vi "Multiple Registration - Unregister.vi"() -> ()   [LabVIEW 2011]
panel:
  in  "Unregister 3":bool
  in  "Unregister 1":bool
  out "Iteration Count #3":i32
  out "Iteration Count #2":i32
  out "Iteration Count #1":i32
  in  "Unregister 2":bool
  out "Process 3 Event #":i32
  out "Process 2 Event #":i32
  out "Process 1 Event #":i32
  in  "Generate Event":bool
  out "Time Process 3 was Stopped":timestamp
  out "Process 3":timestamp
  out "Time Process 2 was Stopped":timestamp
  out "Process 2":timestamp
  out "Time Process 1 was Stopped":timestamp
  in  "stop":bool
  out "Process 1":timestamp
  # "Loop\nIteration\nCount"
  # "Event\nNumber"
  # "User Event Data"
  # "Time Process was stopped"
  # "Process 1"
  # "Process 2"
  # "Process 3"
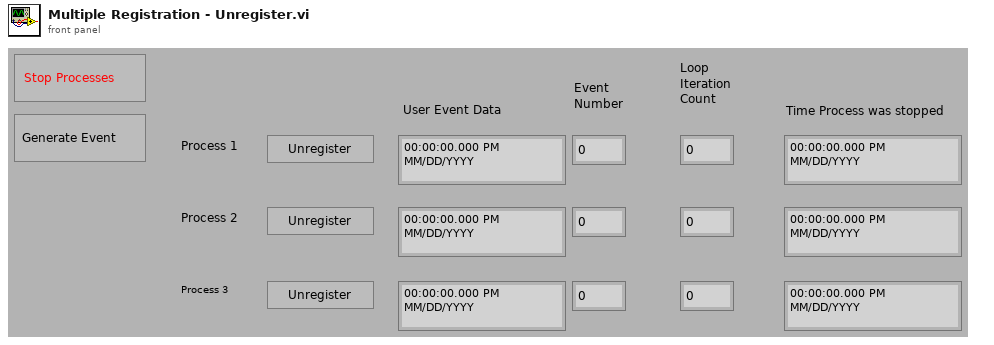
[diagram p1: front panel]
types:
  T1 = cluster{"Event Number":i32, "Event Time":timestamp}
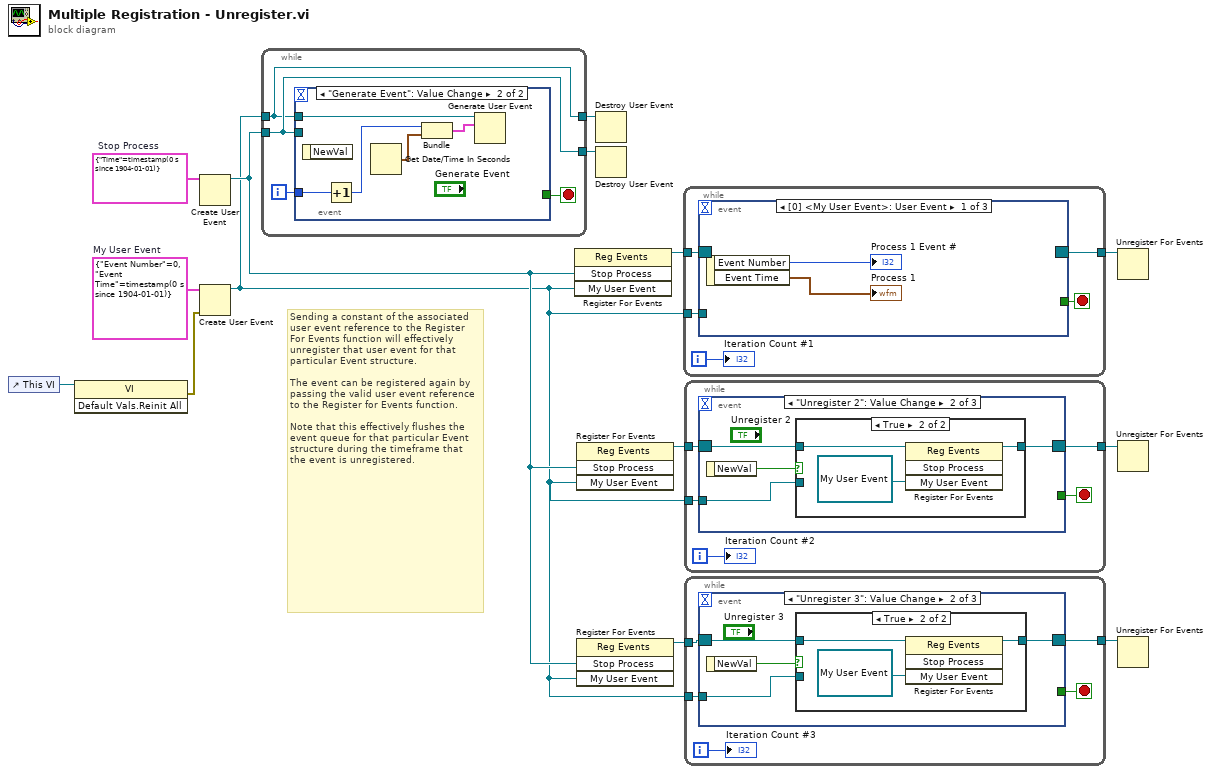
[diagram p0: block diagram]
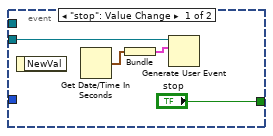
[diagram p2: hidden frame]
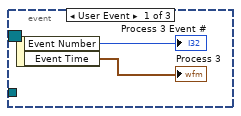
[diagram p3: hidden frame]
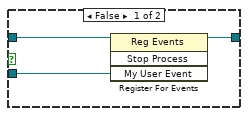
[diagram p4: hidden frame]
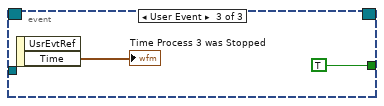
[diagram p5: hidden frame]
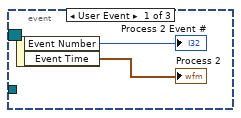
[diagram p6: hidden frame]
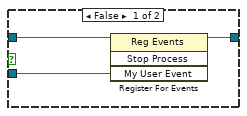
[diagram p7: hidden frame]
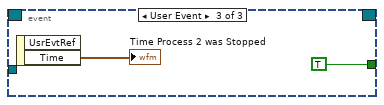
[diagram p8: hidden frame]
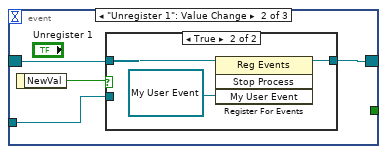
[diagram p9: hidden frame]
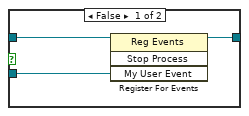
[diagram p10: hidden frame]
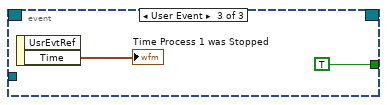
[diagram p11: hidden frame]
diagram:
  w9 = T1 {"Event Number"=0, "Event Time"=timestamp(0 s since 1904-01-01)}  # My User Event
  w14 = cluster{"Time":timestamp} {"Time"=timestamp(0 s since 1904-01-01)}  # Stop Process
  # "Sending a constant of the associated user event reference to the Register For Events function will effectively unregister that user event for that particular Event structure.\n\nThe event can be registered again by passing the valid user event reference to the Register for Events function.\n\nNote that this effectively flushes the event queue for that particular Event structure during the timeframe that the event is unregistered."
  n1 = control-ref of="This VI"() -> (w2:refnum<vi>)
  n2 = invoke class="VI" method="Default Vals.Reinit All"(reference=w2) -> (error out=w1:errorcluster)  [unwired: 2 in, 2 out]
  n3 = Create User Event(user event datatype=w14) -> (user event=w10:refnum<user-event>)  [unwired: 1 in, 1 out]
  n4 = Create User Event(user event datatype=w9, error in=w1) -> (user event=w8:refnum<user-event>)  [unwired: 1 out]
  n5 = while {
    tunnel: w10 -> [w16]
    tunnel: w8 -> [w15]
    tunnel: [w15] -> w7
    tunnel: [w16] -> w6
    i -> [w17]
    stop <- w18 stop-if-true
    n6 = event shown="[1] \"Generate Event\": Value Change" {
      selector: _ -> [_ _]
      dyn-events: _ -> [_ _]
      timeout: _ -> [_ _]
      tunnel: w16 -> [w22 _]
      tunnel: ["stop" _] -> w18
      tunnel: w15 -> [_ w27]
      tunnel: w17 -> [_ w26]
      event "stop": Value Change {
        n7 = event-data() -> ()  [unwired: 1 in, 1 out]
        n8 = Get Date/Time In Seconds() -> (seconds since 1Jan1904=w21:timestamp)
        n9 = Bundle("seconds since 1Jan1904"=w21) -> (w20:cluster{"seconds since 1Jan1904":timestamp})  [unwired: 1 in]
        n10 = Generate User Event(user event=w22, event data cluster=w20) -> ()  [unwired: 1 in, 2 out]
      }
      event "Generate Event": Value Change {
        n11 = event-data() -> ()  [unwired: 1 in, 1 out]
        n12 = Increment(x=w26) -> (x+1=w23:i32)
        n13 = Get Date/Time In Seconds() -> (seconds since 1Jan1904=w25:timestamp)
        n14 = Bundle(w23, "seconds since 1Jan1904"=w25) -> (w24:cluster{i32, "seconds since 1Jan1904":timestamp})  [unwired: 1 in]
        n15 = Generate User Event(user event=w27, event data cluster=w24) -> ()  [unwired: 1 in, 2 out]
      }
    }
  }
  n16 = register-events(w10, w8) -> (reference out=w13:refnum<event-registration>)  [unwired: 2 in, 1 out]
  n17 = register-events(w10, w8) -> (reference out=w12:refnum<event-registration>)  [unwired: 2 in, 1 out]
  n18 = register-events(w10, w8) -> (reference out=w11:refnum<event-registration>)  [unwired: 2 in, 1 out]
  n19 = Destroy User Event(user event=w7) -> ()  [unwired: 1 in, 1 out]
  n20 = Destroy User Event(user event=w6) -> ()  [unwired: 1 in, 1 out]
  n21 = while {
    tunnel: w13 -> [w32]
    tunnel: w8 -> [w29]
    tunnel: [w28] -> w5
    i -> [w30]
    stop <- w31 stop-if-true
    n22 = event shown="[0] <My User Event>: User Event" {
      selector: w32 -> [_ w37 _]
      dyn-events: [_ w36 _] -> w28
      timeout: _ -> [_ _ _]
      tunnel: [_ _ TRUE] -> w31
      tunnel: w29 -> [_ w38 _]
      event User Event {
        n23 = event-data() -> ("Event Number"=→"Process 1 Event #":i32, "Event Time"=→"Process 1":timestamp)  [unwired: 1 in]
      }
      event "Unregister 1": Value Change {
        n24 = event-data() -> ("NewVal"=w35:bool)  [unwired: 1 in]
        n25 = case shown="True" w35 {
          tunnel: w37 -> [w39 w44]
          tunnel: w38 -> [w41 _]
          tunnel: [w40 w43] -> w36
          frame False {
            n26 = register-events(reference=w39, w41) -> (reference out=w40:refnum<event-registration>)  [unwired: 2 in, 1 out]
          }
          frame True {
            n27 = register-events(reference=w44, refnum<user-event> refnum ("event source")) -> (reference out=w43:refnum<event-registration>)  [unwired: 2 in, 1 out]
          }
        }
      }
      event User Event {
        n28 = event-data() -> ("Time"=→"Time Process 1 was Stopped":timestamp)  [unwired: 1 in, 1 out]
      }
    }
    "Iteration Count #1" <- w30
  }
  n29 = while {
    tunnel: w12 -> [w51]
    tunnel: w8 -> [w49]
    tunnel: [w47] -> w4
    i -> [w48]
    stop <- w50 stop-if-true
    n30 = event shown="[1] \"Unregister 2\": Value Change" {
      selector: w51 -> [_ w57 _]
      dyn-events: [_ w54 _] -> w47
      timeout: _ -> [_ _ _]
      tunnel: [_ _ TRUE] -> w50
      tunnel: w49 -> [_ w55 _]
      event User Event {
        n31 = event-data() -> ("Event Number"=→"Process 2 Event #":i32, "Event Time"=→"Process 2":timestamp)  [unwired: 1 in]
      }
      event "Unregister 2": Value Change {
        n32 = event-data() -> ("NewVal"=w56:bool)  [unwired: 1 in]
        n33 = case shown="True" w56 {
          tunnel: w57 -> [w58 w63]
          tunnel: w55 -> [w60 _]
          tunnel: [w59 w62] -> w54
          frame False {
            n34 = register-events(reference=w58, w60) -> (reference out=w59:refnum<event-registration>)  [unwired: 2 in, 1 out]
          }
          frame True {
            n35 = register-events(reference=w63, refnum<user-event> refnum ("event source")) -> (reference out=w62:refnum<event-registration>)  [unwired: 2 in, 1 out]
          }
        }
      }
      event User Event {
        n36 = event-data() -> ("Time"=→"Time Process 2 was Stopped":timestamp)  [unwired: 1 in, 1 out]
      }
    }
    "Iteration Count #2" <- w48
  }
  n37 = while {
    tunnel: w11 -> [w70]
    tunnel: w8 -> [w67]
    tunnel: [w66] -> w3
    i -> [w68]
    stop <- w69 stop-if-true
    n38 = event shown="[1] \"Unregister 3\": Value Change" {
      selector: w70 -> [_ w75 _]
      dyn-events: [_ w74 _] -> w66
      timeout: _ -> [_ _ _]
      tunnel: [_ _ TRUE] -> w69
      tunnel: w67 -> [_ w73 _]
      event User Event {
        n39 = event-data() -> ("Event Number"=→"Process 3 Event #":i32, "Event Time"=→"Process 3":timestamp)  [unwired: 1 in]
      }
      event "Unregister 3": Value Change {
        n40 = event-data() -> ("NewVal"=w76:bool)  [unwired: 1 in]
        n41 = case shown="True" w76 {
          tunnel: w75 -> [w77 w82]
          tunnel: w73 -> [w79 _]
          tunnel: [w78 w81] -> w74
          frame False {
            n42 = register-events(reference=w77, w79) -> (reference out=w78:refnum<event-registration>)  [unwired: 2 in, 1 out]
          }
          frame True {
            n43 = register-events(reference=w82, refnum<user-event> refnum ("event source")) -> (reference out=w81:refnum<event-registration>)  [unwired: 2 in, 1 out]
          }
        }
      }
      event User Event {
        n44 = event-data() -> ("Time"=→"Time Process 3 was Stopped":timestamp)  [unwired: 1 in, 1 out]
      }
    }
    "Iteration Count #3" <- w68
  }
  n45 = Unregister For Events(event registration refnum=w5) -> ()  [unwired: 1 in, 1 out]
  n46 = Unregister For Events(event registration refnum=w4) -> ()  [unwired: 1 in, 1 out]
  n47 = Unregister For Events(event registration refnum=w3) -> ()  [unwired: 1 in, 1 out]
